vi "C1G2_Assemble ACK.vi"(7 "Symbol Rate":dbl=10000000.0 format="%#_6p", 10 "Parameters Select":T2={"Target"=0, "Action"=0, "MemBank"=1, "truncate"=FALSE} {"MemBank" items=["00 RFU", "01 EPC", "10 TID", "11 User"]; "Action" items=["000", "001", "010", "011", "100", "101", "110", "111"]; "Target" items=["000 Inventoried (S0)", "001 Inventoried (S1)", "010 Inventoried (S2)", "011 Inventoried (S3)", "100 SL", "101 RFU", "110 RFU", "111 RFU"]}, 11 "Parameters Symbols":T1={"Tari"=2.5e-05, "PW"=0.5, "factor for \"1\" symbol"=0.5, "RTcal"=2.5, "TRcal"=2.5, "Delimiter"=1.25e-05} {"TRcal" min=1.1 max=3.0 step=0.1; "RTcal" min=2.5 max=3.0 step=0.1; "factor for \"1\" symbol" min=0.5 max=1.0 step=0.1; "PW" min=0.265 max=0.525 step=0.001; "Tari" format="%#_3p"}) -> (2 "Signal out":u8[](array[numeric]))   [LabVIEW 2015]
panel:
  out "Sym0":i32
  out "Sym1":i32
  out "Symbols":i32=53374
  out "Digital Waveform":waveform(u8)(graph)={"t0"=timestamp(0 s since 1904-01-01), "dt"=1e-07, "Y"=array[53374 elements]}
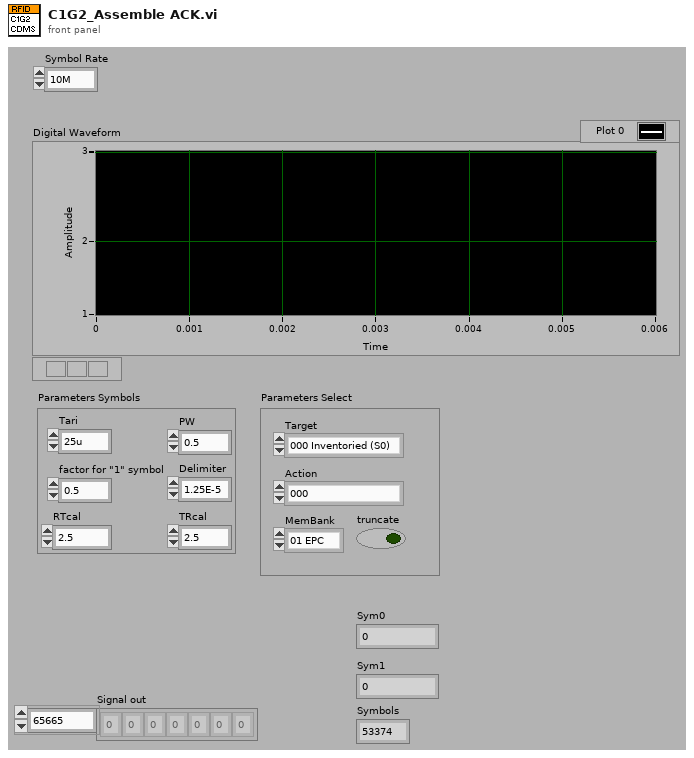
[diagram p1: front panel]
types:
  T1 = cluster{"Tari":dbl, "PW":dbl, "factor for \"1\" symbol":dbl, "RTcal":dbl, "TRcal":dbl, "Delimiter":dbl}
  T2 = cluster{"Target":u16, "Action":u16, "MemBank":u16, "truncate":bool}
  T3 = typedef "C1G2_BasicsData.ctl" = cluster{"Symbol \"0\"":u8[], "Symbol \"1\"":u8[], "RT Preamble":u8[], "RT Frame Sync":u8[], "Sample Rate":dbl, "LOW-Pulse":u8[], "HIGH-Pulse":u8[], "RT cal":u8[]}
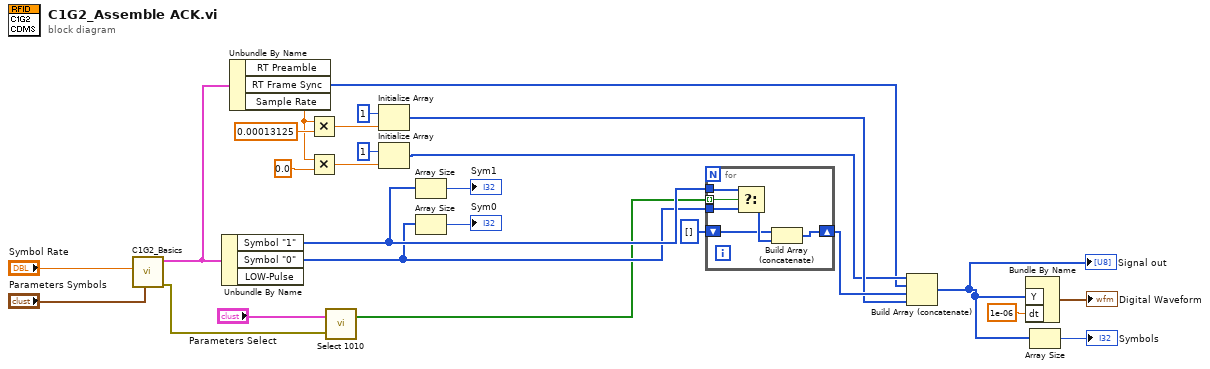
[diagram p0: block diagram]
diagram:
  n1 = call "C1G2_Basics.vi"("Parameters Symbols"="Parameters Symbols", "Symbol Rate"="Symbol Rate") -> ("error out"=w12:errorcluster, "Basic Components"=w13:T3)  [unwired: 8 in]
  n2 = Unbundle By Name(w13) -> ("Symbol \"1\""=w10:u8[], "Symbol \"0\""=w8:u8[])  [unwired: 1 out]
  n3 = Unbundle By Name(w13) -> ("RT Frame Sync"=w3:u8[], "Sample Rate"=w7:dbl)  [unwired: 1 out]
  n4 = Multiply(x=w7, y=0.00013125 ("Pause length /s")) -> (x*y=w19:dbl)
  n5 = Multiply(x=w7, y=0.0 ("Pause length /s")) -> (x*y=w15:dbl)
  n6 = call "Select 1010.vi"("error in (no error)"=w12, "Parameters Select"="Parameters Select") -> ("Array"=w1:bool[])  [unwired: 1 out]
  n7 = Initialize Array(u8 1 ("element"), w19) -> (w5:u8[])
  n8 = Initialize Array(u8 1 ("element"), w15) -> (w4:u8[])
  n9 = Array Size(array=w10) -> (size(s)=→"Sym1":i32)
  n10 = Array Size(array=w8) -> (size(s)=→"Sym0":i32)
  n11 = for {
    tunnel: w8 -> [w31]
    tunnel: w10 -> [w32]
    shift-right: [w30] -> w6
    shift-left: u8[] [] ("s? t:f") -> [w28]
    tunnel: w1 -> [w27] mode=indexing
    n12 = Select(t=w32, s=w27, f=w31) -> (s? t:f=w29:u8[])
    n13 = Build Array (concatenate)(w28, w29) -> (w30:u8[])
  }
  n14 = Build Array (concatenate)(w4, w3, w6, w5) -> (w2:u8[])
  "Signal out" <- w2
  n15 = Bundle By Name("Y"=w2, "dt"=1e-06) -> (→"Digital Waveform":waveform(u8))  [unwired: 1 in]
  n16 = Array Size(array=w2) -> (size(s)=→"Symbols":i32)
